vi "Ex13 Object Tracking PRJ.vi"() -> ()   [LabVIEW 2024]
panel:
  out "error out":errorcluster
  out "RGB IMG":T1(plugin-control)
  out "Circles Data (calibrated)":T2(array[cluster])
  out "BINARY IMG":T1(plugin-control)
  in  "Stop (F)":bool
  # "EX.13 OBJECT TRACKING PRJ"
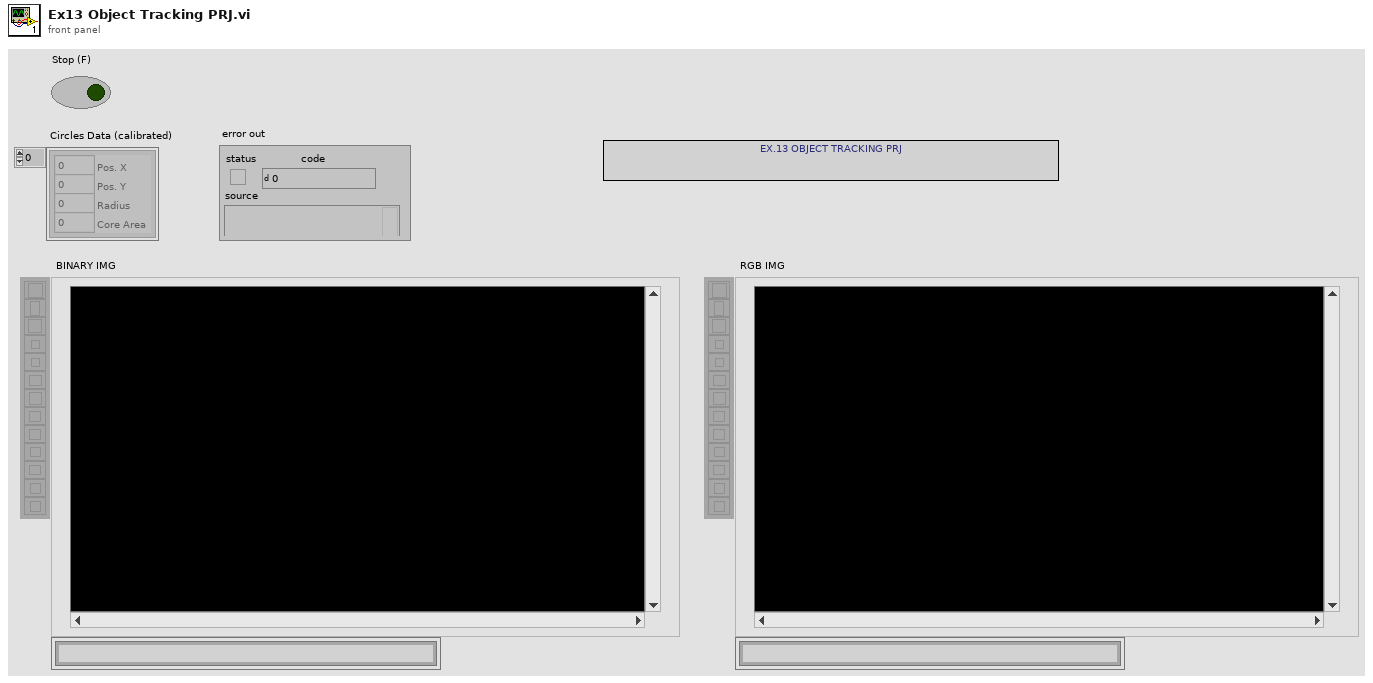
[diagram p1: front panel]
types:
  T1 = typedef "IMAQ Image.ctl" = refnum<image>
  T2 = cluster{"Pos. X":i32, "Pos. Y":i32, "Radius":i32, "Core Area":i32}[]
  T3 = cluster{"Pos. X":i32, "Pos. Y":i32, "Radius":i32, "Core Area":i32}
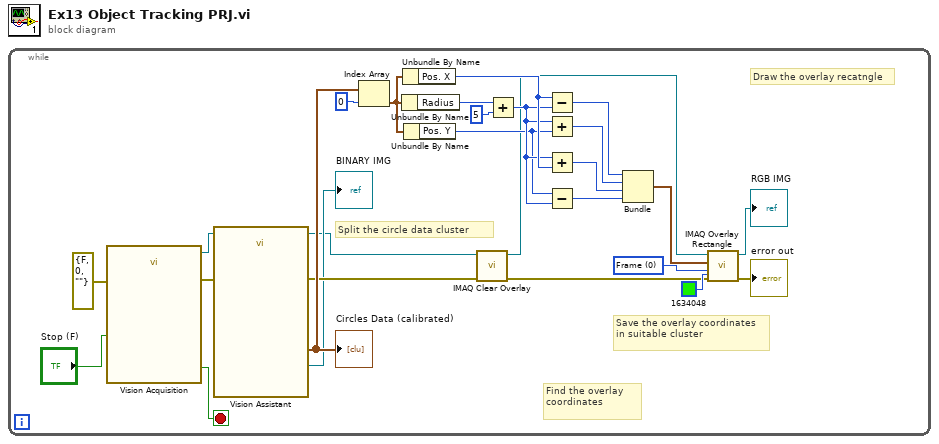
[diagram p0: block diagram]
diagram:
  n1 = while {
    stop <- w25 stop-if-true
    w21 = u32 0 items=["Frame", "Fill", "Highlight"] ("Drawing Mode (Frame)")
    # "Draw the overlay recatngle"
    # "Save the overlay coordinates in suitable cluster"
    # "Find the overlay coordinates"
    # "Split the circle data cluster"
    n2 = call "Vision Acquisition"("Stop (F)"="Stop (F)", "error in"=errorcluster {"status"=FALSE, "code"=0, "source"=""}) -> ("Image Out"=w26:T1, "Stopped"=w25:bool, "error out"=w7:errorcluster)  [unwired: 22 in, 1 out]
    n3 = call "Vision Assistant"("Image In"=w26, "error in"=w7) -> ("Image Out"=w1:T1, "Circles Data (calibrated) (Circle Detection 1)"=w24:T2, "Image Buffer (Image Buffer 4)"=→"BINARY IMG":T1, "error out"=w5:errorcluster)  [unwired: 20 in, 2 out]
    "Circles Data (calibrated)" <- w24
    n4 = Index Array(array=w24, index=0) -> (element=w22:T3)
    n5 = Unbundle By Name(w22) -> ("Radius"=w20:i32)
    n6 = Unbundle By Name(w22) -> ("Pos. X"=w18:i32)
    n7 = Unbundle By Name(w22) -> ("Pos. Y"=w16:i32)
    n8 = call "IMAQ Clear Overlay"("error in (no error)"=w5, "Image"=w1) -> ("error out"=w4:errorcluster, "Image Out"=w3:T1)  [unwired: 8 in]
    n9 = Add(x=w20, y=5) -> (x+y=w17:i32)
    n10 = Subtract(x=w18, y=w17) -> (x-y=w15:i32)
    n11 = Add(x=w17, y=w16) -> (x+y=w14:i32)
    n12 = Add(x=w17, y=w18) -> (x+y=w12:i32)
    n13 = Subtract(x=w16, y=w17) -> (x-y=w11:i32)
    n14 = Bundle(w15, w14, w12, w11) -> (w13:cluster{i32, i32, i32, i32})  [unwired: 1 in]
    n15 = call "IMAQ Overlay Rectangle"("Color"=u32 1634048, "error in (no error)"=w4, "Drawing Mode (Frame)"=w21, "Rectangle"=w13, "Image"=w3) -> ("error out"=→"error out":errorcluster, "Image Out"=→"RGB IMG":T1)  [unwired: 5 in]
  }
